vi "Tacking Helper - Starting Angle Determination.vi"(6 "Boat <> 2nd wp Angle":dbl, 7 "Is the boat to wp\nangle greater than 0?":bool, 9 "Max Angle\nof Tack":dbl, 10 "Min Angle\nof Tack":dbl, 11 "Angle from boat to waypoint":dbl) -> (2 "Second Angle":dbl, 3 "Starting Angle":dbl)   [LabVIEW 2011]
doc: "This vi takes in the current waypoint and the secondary waypoint, and determines whether we should approach right or approach left (whichever one will make us head towards the second waypoint) and then sets the correct starting angle from the min/max tack values.\n\nThe boolean test is necessary because you have to do a different test depending on whether the 'boat to wp' angle is greater or less than 0 (on a -pi tp pi scale) at least with the approach I used."
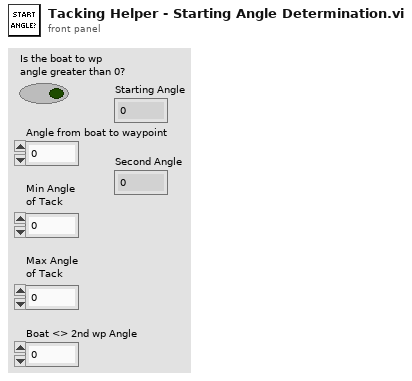
[diagram p1: front panel]
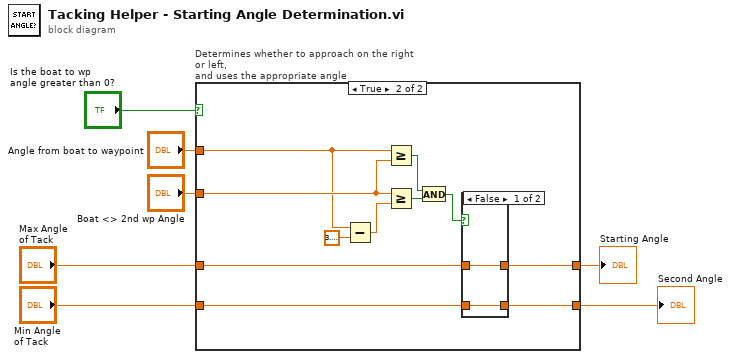
[diagram p0: block diagram]
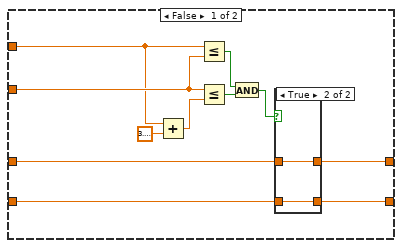
[diagram p2: hidden frame]
diagram:
  n1 = case "Determines whether to approach on the right or left,\nand uses the appropriate angle" shown="True" "Is the boat to wp\nangle greater than 0?" {
    tunnel: "Angle from boat to waypoint" -> [w13 w30]
    tunnel: "Boat <> 2nd wp Angle" -> [w14 w32]
    tunnel: "Max Angle\nof Tack" -> [w11 w26]
    tunnel: "Min Angle\nof Tack" -> [w10 w25]
    tunnel: [w9 w24] -> w6
    tunnel: [w8 w23] -> w7
    frame False {
      n2 = Add(x=w13, y=3.141592653589793) -> (x+y=w16:dbl)
      n3 = Less Or Equal?(x=w13, y=w14) -> (x <= y?=w18:bool)
      n4 = Less Or Equal?(x=w14, y=w16) -> (x <= y?=w15:bool)
      n5 = And(x=w18, y=w15) -> (x .and. y?=w12:bool)
      n6 = case shown="True" w12 {
        tunnel: w11 -> [w20 w21]
        tunnel: w10 -> [w19 w22]
        tunnel: [w19 w21] -> w9
        tunnel: [w20 w22] -> w8
        frame False {
        }
        frame True {
        }
      }
    }
    frame True {
      n7 = Subtract(x=w30, y=3.141592653589793) -> (x-y=w29:dbl)
      n8 = Greater Or Equal?(x=w30, y=w32) -> (x >= y?=w33:bool)
      n9 = Greater Or Equal?(x=w32, y=w29) -> (x >= y?=w28:bool)
      n10 = And(x=w33, y=w28) -> (x .and. y?=w27:bool)
      n11 = case shown="False" w27 {
        tunnel: w26 -> [w35 w36]
        tunnel: w25 -> [w34 w37]
        tunnel: [w34 w36] -> w23
        tunnel: [w35 w37] -> w24
        frame False {
        }
        frame True {
        }
      }
    }
  }
  "Second Angle" <- w7
  "Starting Angle" <- w6
